vi "AgilentTriggered.vi"() -> ()   [LabVIEW 2014]
uses:
  <vilib>/Utility/error.llb/DialogType.ctl
  <instrlib>/Agilent 34401/Agilent 34401.lvlib
panel:
  in  "Manual Resolution (5.5 Digits)":dbl(ring)=5.5 items=["4.5"=4.5, "5.5"=5.5, "6.5"=6.5]
  in  "Slope (0: Negative)":u16(ring)=1 items=["Negative", "Positive"]
  in  "Function (0: DC Voltage)":u16(ring) items=["DC Voltage", "AC Voltage", "2 - Wire Resistance", "4 - Wire Resistance", "DC Current", "AC Current", "Frequency", "Period", "Continuity", "Diode Checking", "VDC:VDC Ratio", "Temperature", "Capacitance"]
  in  "Trigger Source (0: Immediate)":u16(ring)=2 items=["Immediate", "Software (Bus)", "External", "Internal"]
  in  "Manual Range (1.00)":dbl=10.0 format="%_3f"
  in  "Enable Auto Range (F: Disable)":bool
  in  "Trigger Count (5)":i32=5 format="%#.6g"
  out "Measurements":dbl[](graph)=[0.002500734, 0.002496723, 0.002491019, 0.002484271, 0.002477294]
  out "Trigger Iteration":i32
  in  "Stop":bool
  in  "Samples per Trigger (10)":i32=1 format="%#.6g"
  in  "Timeout (10000 ms)":u32=40000
  in  "VISA resource name":refnum<visa-resource-name>
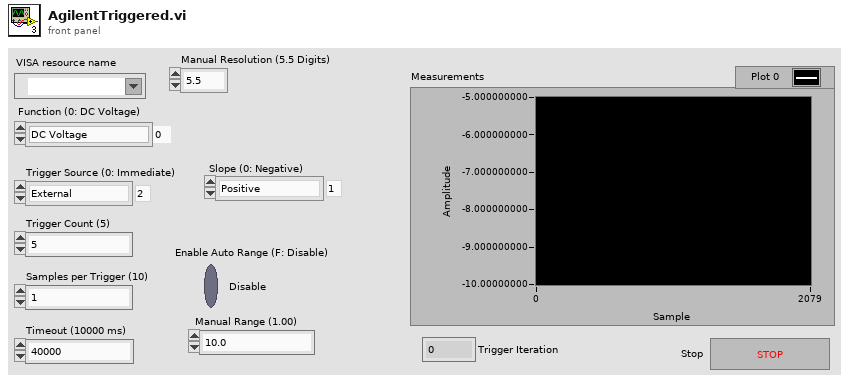
[diagram p1: front panel]
types:
  T1 = typedef "DialogType.ctl" = u16
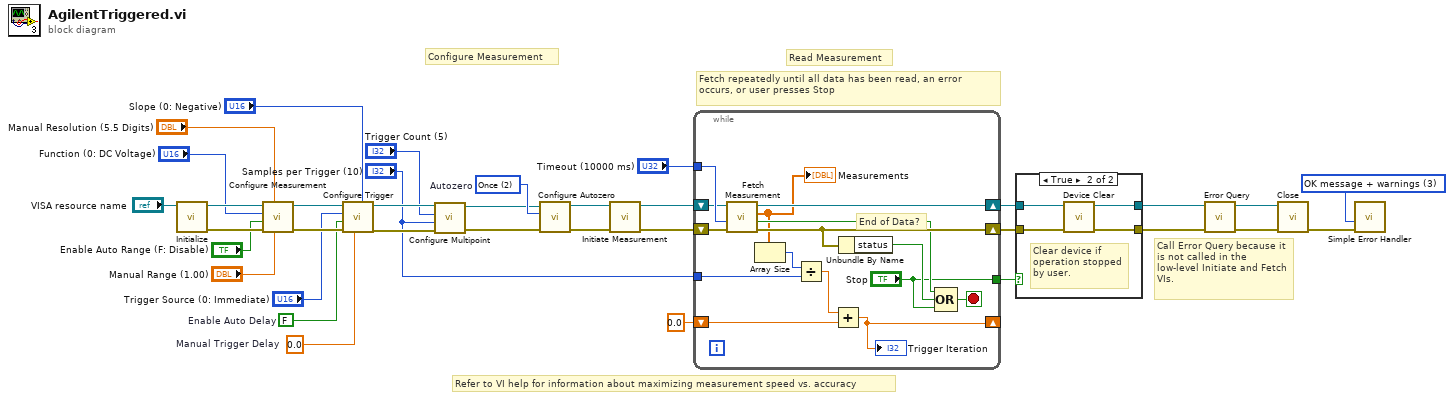
[diagram p0: block diagram]
diagram:
  w4 = 0.0  # Manual Trigger Delay
  w5 = FALSE  # Enable Auto Delay
  w13 = T1 3 items=["no dialog", "OK message", "continue or stop message", "OK message + warnings", "continue/stop + warnings"] ("type of dialog (OK msg:1)")
  w31 = u16 2 items=["On", "Off", "Once"]  # Autozero
  # "Call Error Query because it is not called in the low-level Initiate and Fetch VIs."
  # "Fetch repeatedly until all data has been read, an error occurs, or user presses Stop"
  # "Refer to VI help for information about maximizing measurement speed vs. accuracy"
  # "Read Measurement"
  # "Configure Measurement"
  n1 = call <instrlib>:"Initialize.vi"("VISA resource name"="VISA resource name") -> ("error out"=w32:errorcluster, "VISA resource name out"=w33:refnum<visa-resource-name>)  [unwired: 9 in]
  n2 = call <instrlib>:"Configure Measurement.vi"("Manual Range (1.00)"="Manual Range (1.00)", "Manual Resolution (5.5 Digits)"="Manual Resolution (5.5 Digits)", "error in (no error)"=w32, "Enable Auto Range (T: Enable)"="Enable Auto Range (F: Disable)", "Function (0: DC Voltage)"="Function (0: DC Voltage)", "VISA resource name"=w33) -> ("error out"=w24:errorcluster, "VISA resource name out"=w25:refnum<visa-resource-name>)  [unwired: 4 in]
  n3 = call <instrlib>:"Configure Trigger.vi"("Slope (0: Negative)"="Slope (0: Negative)", "Manual Trigger Delay (0.0 s)"=w4, "error in (no error)"=w24, "Enable Auto Delay (T: Enable)"=w5, "Trigger Source (0: Immediate)"="Trigger Source (0: Immediate)", "VISA resource name"=w25) -> ("error out"=w22:errorcluster, "VISA resource name out"=w23:refnum<visa-resource-name>)  [unwired: 4 in]
  n4 = call <instrlib>:"Configure Multipoint.vi"("error in (no error)"=w22, "Sample Count (1)"="Samples per Trigger (10)", "Trigger Count (1)"="Trigger Count (5)", "VISA resource name"=w23) -> ("error out"=w28:errorcluster, "VISA resource name out"=w29:refnum<visa-resource-name>)  [unwired: 6 in]
  n5 = call <instrlib>:"Configure Autozero.vi"("error in (no error)"=w28, "Autozero  (0: On)"=w31, "VISA resource name"=w29) -> ("error out"=w20:errorcluster, "VISA resource name out"=w21:refnum<visa-resource-name>)  [unwired: 7 in]
  n6 = call <instrlib>:"Initiate Measurement.vi"("error in (no error)"=w20, "VISA resource name"=w21) -> ("error out"=w18:errorcluster, "VISA resource name out"=w19:refnum<visa-resource-name>)  [unwired: 8 in]
  n7 = while {
    tunnel: "Timeout (10000 ms)" -> [w49]
    shift-right: [w45] -> w26
    shift-left: w18 -> [w47]
    shift-right: [w50] -> w27
    shift-left: w19 -> [w48]
    tunnel: ["Stop"] -> w17
    tunnel: "Samples per Trigger (10)" -> [w39]
    shift-right: [w37] -> _
    shift-left: 0.0 -> [w36]
    stop <- w46 stop-if-true
    # "End of Data?"
    n8 = call <instrlib>:"Fetch Measurement.vi"("error in (no error)"=w47, "Timeout (10000 ms)"=w49, "VISA resource name"=w48) -> ("error out"=w45:errorcluster, "End of Data?"=w43:bool, "Measurements"=w41:dbl[], "VISA resource name out"=w50:refnum<visa-resource-name>)  [unwired: 5 in]
    "Measurements" <- w41
    n9 = Array Size(array=w41) -> (size(s)=w40:i32)
    n10 = Divide(x=w40, y=w39) -> (x/y=w38:dbl)
    n11 = Add(x=w38, y=w36) -> (x+y=w37:dbl)
    "Trigger Iteration" <- w37
    n12 = Unbundle By Name(w45) -> ("status"=w44:bool)
    n13 = Compound Arithmetic op=OR(w43, w44, "Stop") -> (w46:bool)
  }
  n14 = case shown="True" w17 {
    tunnel: w27 -> [w52 w56]
    tunnel: w26 -> [w51 w55]
    tunnel: [w52 w54] -> w8
    tunnel: [w51 w53] -> w7
    frame False {
    }
    frame True {
      # "Clear device if operation stopped by user."
      n15 = call <instrlib>:"Device Clear.vi"("error in (no error)"=w55, "VISA Resource Name"=w56) -> ("error out"=w53:errorcluster, "VISA Resource Out"=w54:refnum<visa-resource-name>)  [unwired: 8 in]
    }
  }
  n16 = call <instrlib>:"Error Query.vi"("error in (no error)"=w7, "VISA resource name"=w8) -> ("error out"=w10:errorcluster, "VISA resource name out"=w9:refnum<visa-resource-name>)  [unwired: 6 in, 2 out]
  n17 = call <instrlib>:"Close.vi"("error in (no error)"=w10, "VISA resource name"=w9) -> ("error out"=w35:errorcluster)  [unwired: 9 in]
  n18 = call <vilib>:"Simple Error Handler.vi"("type of dialog (OK msg:1)"=w13, "error in (no error)"=w35) -> ()  [unwired: 3 in, 5 out]
